vi "MM6.ProcCases.vi"(0 "i ref in":refnum<vi>, 1 "selector":string, 2 "Data":T1, 3 "call cluster":T3={"Object"="", "Selector"="", "CallType"=enum."synchronous", "Async Object"="", "Async Selector"="", "Data Descriptor"="", "Data"=[], "Error #"=0, "Expire"=0}, 5 "error in (no error)":errorcluster) -> (14 "i ref out":refnum<vi>, 17 "answer cluster":T3={"Object"="", "Selector"="", "CallType"=enum."synchronous", "Async Object"="", "Async Selector"="", "Data Descriptor"="", "Data"=[], "Error #"=0, "Expire"=0}, 19 "error out":errorcluster)   [LabVIEW 2014, in "MM6.lvlib"]
doc: "This method is called by a process from within the default case in the event loop. The methods of a class that are linked to events will be called from THIS method. Add your code here."
uses:
  MM6.lvlib
  CS_Core/CSSystem/CoreDefs/CoreDefs.call_type.ctl
  CS_Core/BaseProcess/BaseProcess.descriptor string definition.ctl
  CS_Core/CSSystem/CoreDefs/CoreDefs.rawDataType.ctl
  MM6.status.ctl
  CS_Core/CSSystem/CoreLib/CoreLib.byte array 2 string.vi
  CS_Core/CSSystem/CoreLib/CoreLib.string 2 byte array.vi
  CS_Core/BaseProcess/BaseProcess.lvlib
  CS_Core/CSSystem/CoreLib/CoreLib.lvlib
  CS_Core/CSSystem/CSSystemLib/CSSystemLib.lvlib
  CSlibraries-extern/DimLVEvent/LVDimInterface/LVDimInterface.lvlib
panel:
  in  "MMStatus":T2=enum."config"
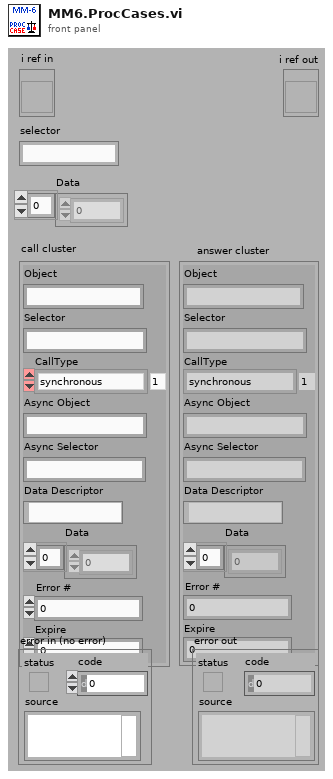
[diagram p1: front panel]
types:
  T1 = typedef "CoreDefs.rawDataType.ctl" = i8[]
  T2 = typedef "MM6.lvlib/MM6.status.ctl" = enum16{"loaded", "load_error", "config", "config_error", "init", "init_error", "data_reset", "data_reset_error", "running", "start_error", "run_error", "abort_requested", "aborted", "stop_requested", "stopped", "stop_error", "Connected", "NOTConnected"}
  T3 = typedef "CoreDefs.call_type.ctl" = cluster{"Object":string, "Selector":string, "CallType":enum16{"simple", "synchronous", "asynchronous"}, "Async Object":string, "Async Selector":string, "Data Descriptor":T4, "Data":T1, "Error #":i32, "Expire":u32}
  T4 = typedef "BaseProcess.lvlib/BaseProcess.descriptor string definition.ctl" = string
  T5 = typedef "MM6.lvlib/MM6.i attribute.ctl" = cluster{"ConfigData":T6, "UsedObjs":string[], "ActScanStep":i32[], "AbortRequest":bool, "StopRequest":bool, "# cycles":i32, "Connected":bool, "MMStatus":T2, "# data":i32, "DIMServices":cluster{"MM6StatusString":string, "MM6StatusID":i32, "discArchiver":string, "discArchiverID":i32, "eventBuilder":string, "eventBuilderID":i32, "GUIIDString":string, "GUIIDStringID":i32}, "dataFile":string, "ExtraDataSets":T21, "PGRunning":T22}
  T6 = typedef "LEBITDefs.lvlib/LEBITDefs.ConfigData.ctl" = cluster{"GenConfig":T7, "Configs":T9[]}
  T7 = typedef "LEBITDefs.lvlib/LEBITDefs.GenConfig.ctl" = cluster{"Mode":i32, "Logs":T8[]}
  T8 = typedef "LEBITDefs.lvlib/LEBITDefs.Log.ctl" = cluster{"Name":string, "FctName":string, "Special":string}
  T9 = typedef "LEBITDefs.lvlib/LEBITDefs.OneConfig.ctl" = cluster{"MCA":T10, "Timing":T11, "Scans":T14[], "FreqDevs":T15[], "CleanDev":T16, "NrCycles":i32, "Specials":T18[], "Delays":T19[], "DAC":T20}
  T10 = typedef "LEBITDefs.lvlib/LEBITDefs.MCA.ctl" = cluster{"Name":string, "Address":string, "NrChannels":i32, "Gate":i32, "NrPipse":i32}
  T11 = typedef "LEBITDefs.lvlib/LEBITDefs.Timing.ctl" = cluster{"TimeTables":cluster{"TimeTable":T12}[], "Memories":T13[], "ScanX":string, "ScanY":string}
  T12 = typedef "LEBITDefs.lvlib/LEBITDefs.Timetable.ctl" = dbl[]
  T13 = typedef "LEBITDefs.lvlib/LEBITDefs.Memory.ctl" = cluster{"Device":string, "ExtTrig":bool, "TT2Use":i32, "PatternTable":string[]}
  T14 = typedef "LEBITDefs.lvlib/LEBITDefs.ScanDev.ctl" = cluster{"Name":string, "FctName":string, "Values":dbl[], "NrScanVals":i32, "Special":string}
  T15 = typedef "LEBITDefs.lvlib/LEBITDefs.FreqDev.ctl" = cluster{"Name":string, "Amp":dbl, "CenterFreq":dbl, "Time":dbl}
  T16 = typedef "LEBITDefs.lvlib/LEBITDefs.CleanDev.ctl" = cluster{"Name":string, "CleanData":T17[]}
  T17 = typedef "LEBITDefs.lvlib/LEBITDefs.CleanDataType.ctl" = cluster{"Amp":dbl, "Center":dbl, "Plus":dbl, "Minus":dbl, "Time":dbl}
  T18 = typedef "LEBITDefs.lvlib/LEBITDefs.Special.ctl" = cluster{"Name":string, "FctName":string, "VerySpecial":string, "Data":dbl}
  T19 = typedef "LEBITDefs.lvlib/LEBITDefs.Delay.ctl" = cluster{"Name":string, "Delay":dbl}
  T20 = typedef "LEBITDefs.lvlib/LEBITDefs.DAC.ctl" = cluster{"Name":string, "Step1":i32, "Step2":i32}
  T21 = typedef "LEBITDefs.lvlib/LEBITDefs.ExtraData.ctl" = cluster{"Ions":cluster{"ExcitIonMass":string, "ExcitIonCharge":i32, "CleanIons":cluster{"CleanIonMass":string, "CleanIonCharge":i32}[]}, "TimingDescription":cluster{"TimeTableDescription":cluster{"Times":string[]}[], "PatternTableDescription":cluster{"Pattern":string[]}[]}, "ScanUnits":string[]}[]
  T22 = typedef "PPG_ABC.lvlib/PPG_ABC.PG_Running.ctl" = i32
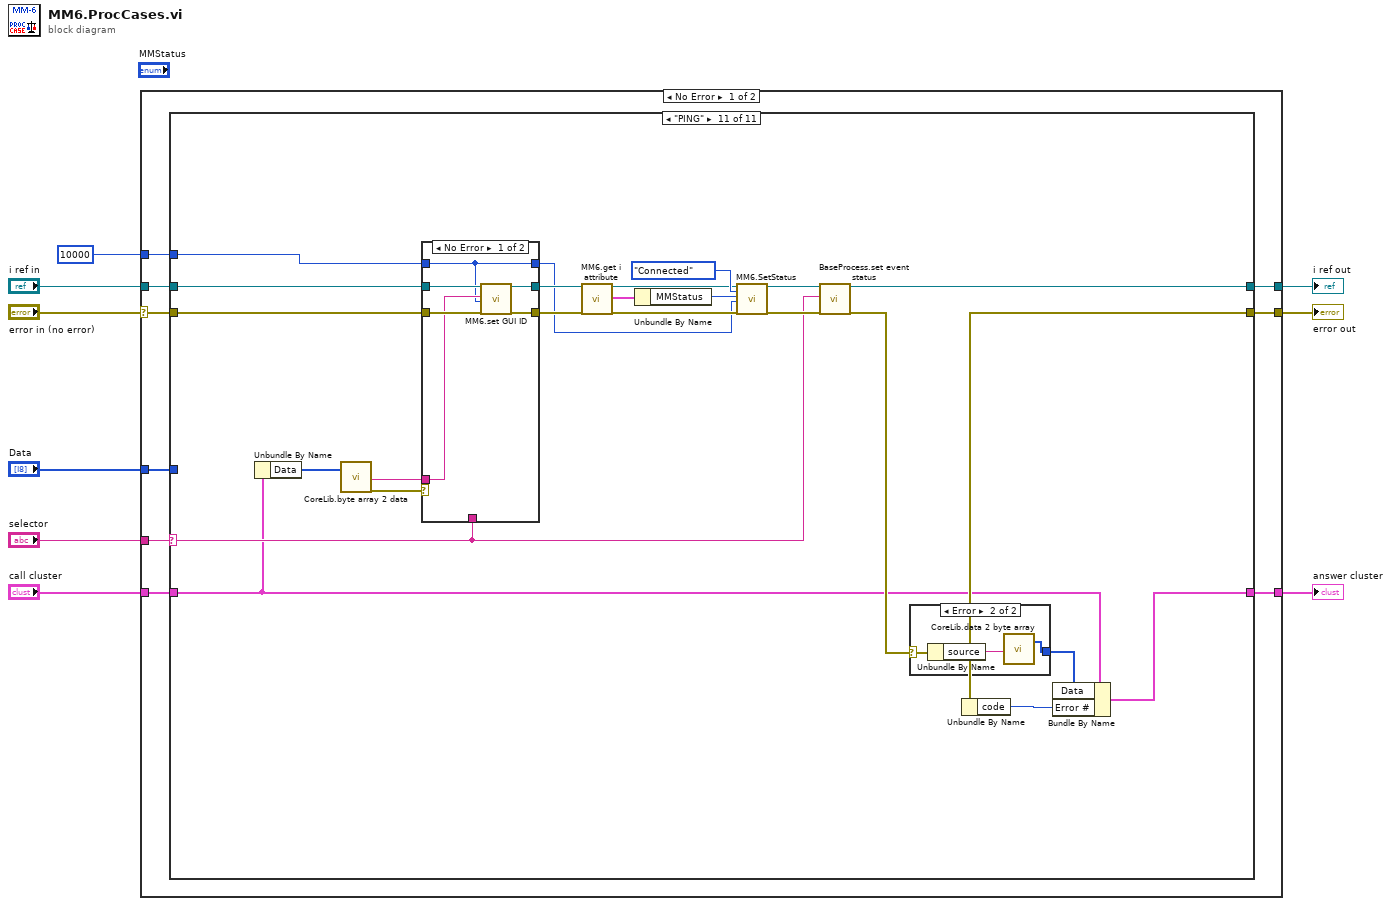
[diagram p0: block diagram]
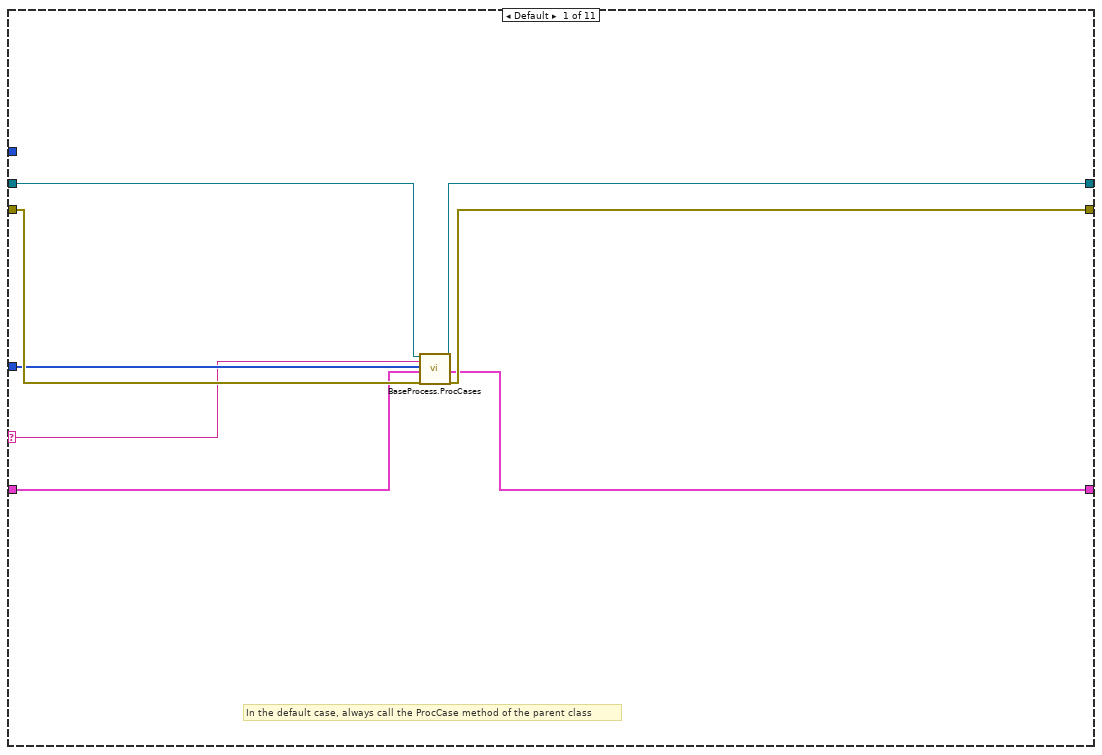
[diagram p2: hidden frame]
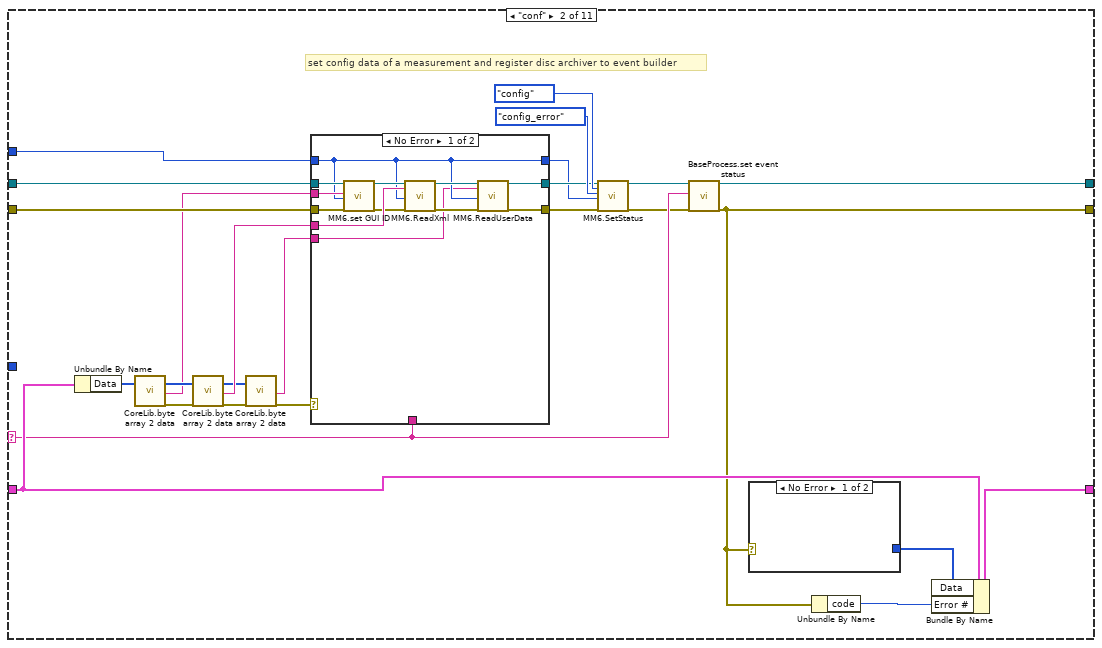
[diagram p3: hidden frame]
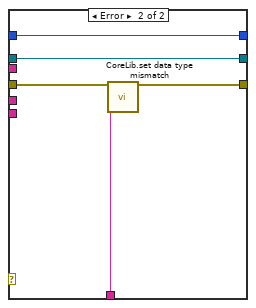
[diagram p4: hidden frame]
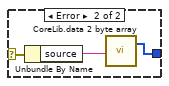
[diagram p5: hidden frame]
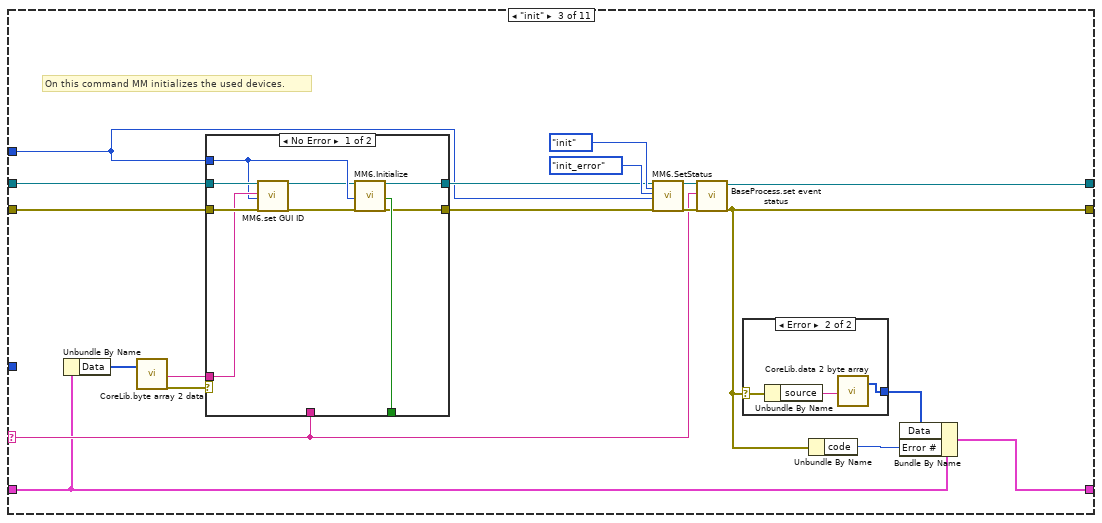
[diagram p6: hidden frame]
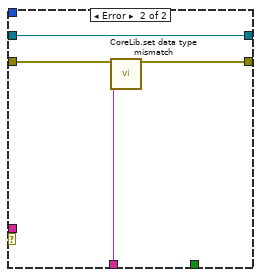
[diagram p7: hidden frame]
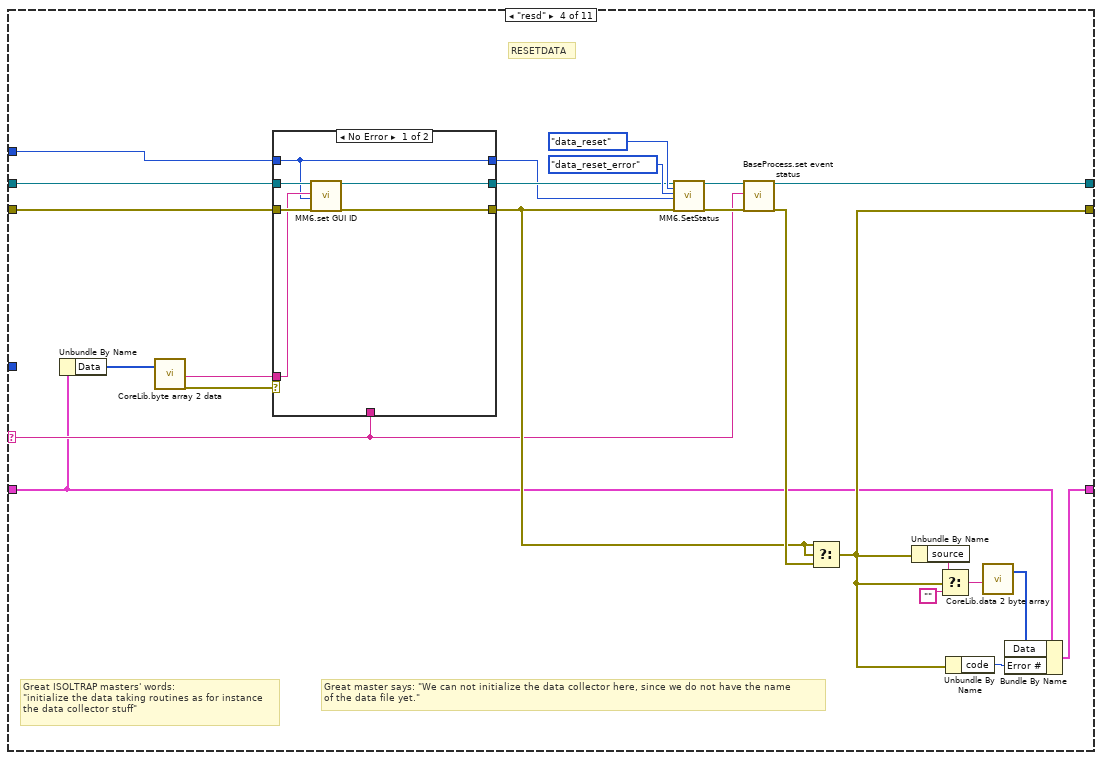
[diagram p9: hidden frame]
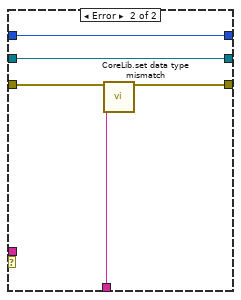
[diagram p10: hidden frame]
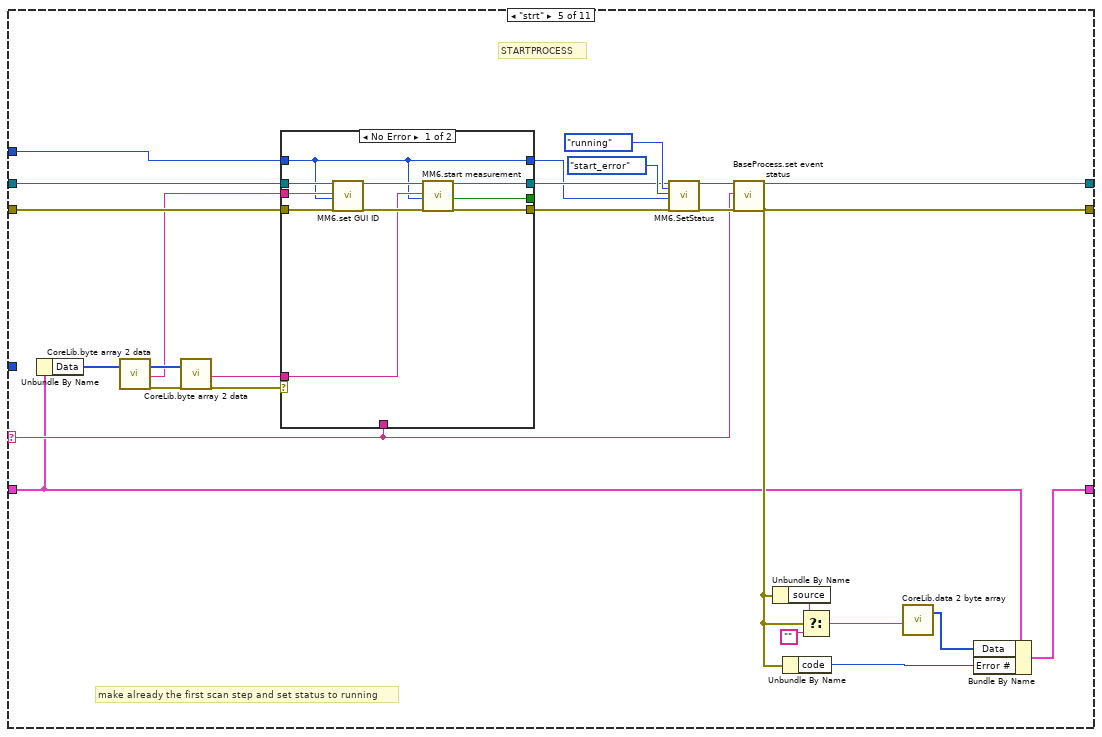
[diagram p11: hidden frame]
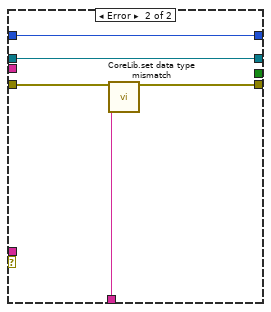
[diagram p12: hidden frame]
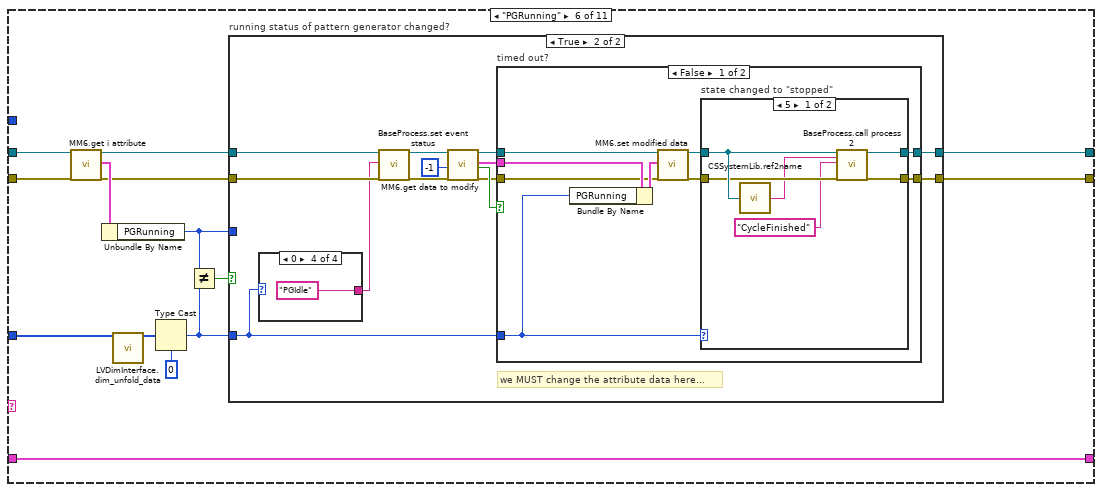
[diagram p13: hidden frame]
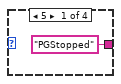
[diagram p15: hidden frame]
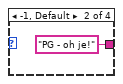
[diagram p16: hidden frame]
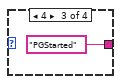
[diagram p17: hidden frame]
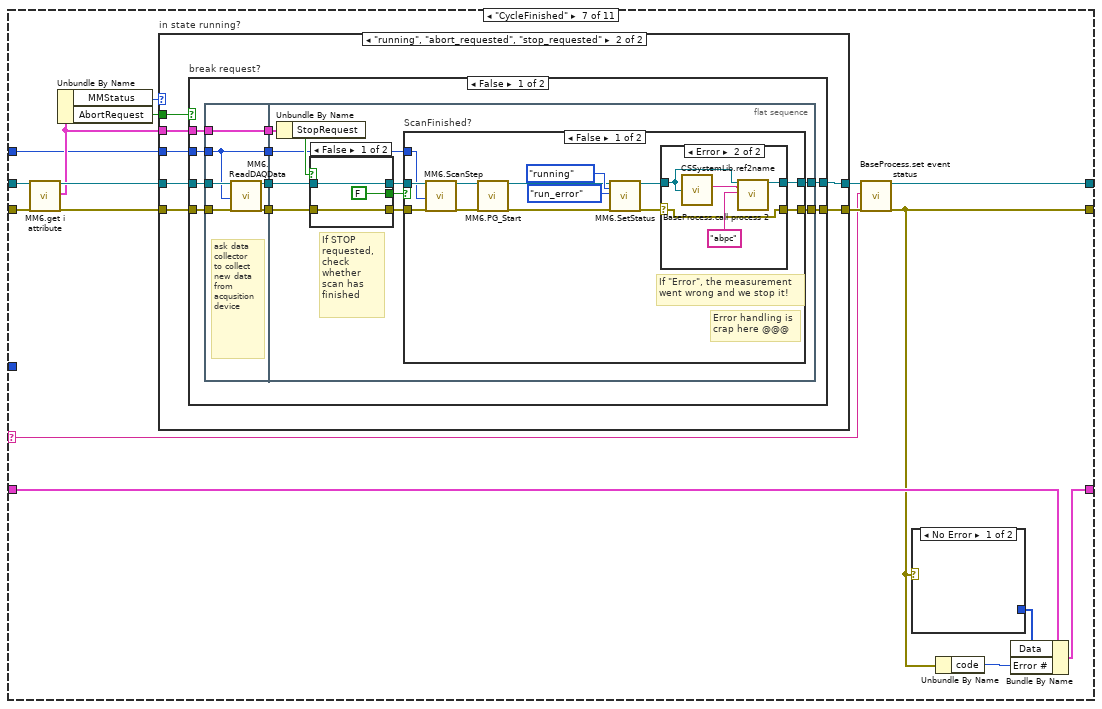
[diagram p20: hidden frame]
diagram:
  n1 = case shown="No Error" "error in (no error)" {
    selector: "error in (no error)" -> [w10 w527]
    tunnel: [w18 w528] -> w9
    tunnel: "call cluster" -> [w17 w528]
    tunnel: [w16 w529] -> w7
    tunnel: [w15 w527] -> w6
    tunnel: "i ref in" -> [w14 w529]
    tunnel: "selector" -> [w13 _]
    tunnel: 10000 ("ms timeout (100)") -> [w12 _]
    tunnel: "Data" -> [w11 _]
    frame No Error {
      n2 = case shown="\"PING\"" w13 {
        selector: w13 -> [w20 w46 w75 w113 w148 _ w237 w338 w398 w450 w492]
        tunnel: w11 -> [w21 _ _ _ _ w197 _ _ _ _ _]
        tunnel: [w26 w41 w81 w129 w168 w186 w241 w354 w413 w469 w512] -> w16
        tunnel: w17 -> [w22 w50 w73 w109 w143 w187 w248 w337 w397 w449 w491]
        tunnel: [w23 w49 w91 w130 w166 w187 w247 w355 w414 w467 w510] -> w18
        tunnel: w10 -> [w25 w32 w78 w114 w153 w193 w251 w358 w417 w454 w497]
        tunnel: [w24 w48 w90 w125 w163 w188 w240 w353 w412 w468 w511] -> w15
        tunnel: w12 -> [_ w36 w80 w112 w151 _ w238 w342 w402 w453 w494]
        tunnel: w14 -> [w19 w33 w79 w116 w155 w194 w252 w359 w418 w455 w500]
        frame Default {
          # "In the default case, always call the ProcCase method of the parent class"
          n3 = call "BaseProcess.ProcCases.vi"("i ref in"=w19, "selector"=w20, "Data"=w21, "call cluster"=w22, "error in (no error)"=w25) -> ("i ref out"=w26:refnum<vi>, "answer cluster"=w23:T3, "error out"=w24:errorcluster)  [unwired: 12 in]
        }
        frame "conf" {
          # "set config data of a measurement and register disc archiver to event builder"
          n4 = Unbundle By Name(w50) -> ("Data"=w47:T1)
          n5 = call-poly "CoreLib.byte array 2 data.vi"("byteArray"=w47) -> ("byteArray out"=w40:T1, "string"=w31:string, "error out"=w39:errorcluster)  [unwired: 16 in]
          n6 = call-poly "CoreLib.byte array 2 data.vi"("byteArray"=w40, "error in (no error)"=w39) -> ("byteArray out"=w29:T1, "string"=w34:string, "error out"=w30:errorcluster)  [unwired: 15 in]
          n7 = call-poly "CoreLib.byte array 2 data.vi"("byteArray"=w29, "error in (no error)"=w30) -> ("string"=w28:string, "error out"=w27:errorcluster)  [unwired: 15 in, 1 out]
          n8 = case shown="No Error" w27 {
            tunnel: [w55 w68] -> w42
            tunnel: w46 -> [_ w69]
            tunnel: w32 -> [w62 w67]
            tunnel: w33 -> [w63 w66]
            tunnel: [w56 w66] -> w37
            tunnel: w36 -> [w54 w65]
            tunnel: [w54 w65] -> w35
            tunnel: w34 -> [w64 _]
            tunnel: w31 -> [w61 _]
            tunnel: w28 -> [w53 _]
            frame No Error {
              n9 = call "MM6.set GUI ID.vi"("i ref in"=w63, "GUIDString"=w61, "ms timeout (10000)"=w54, "error in (no error)"=w62) -> ("i ref out"=w60:refnum<vi>, "error out"=w59:errorcluster)  [unwired: 13 in, 1 out]
              n10 = call "MM6.ReadXml.vi"("i ref in"=w60, "Data"=w64, "timeout ms"=w54, "error in (no error)"=w59) -> ("i ref out"=w58:refnum<vi>, "error out"=w57:errorcluster)  [unwired: 13 in, 1 out]
              n11 = call "MM6.ReadUserData.vi"("i ref in"=w58, "Data"=w53, "timeout ms"=w54, "error in (no error)"=w57) -> ("i ref out"=w56:refnum<vi>, "error out"=w55:errorcluster)  [unwired: 13 in, 1 out]
            }
            frame Error {
              n12 = call "CoreLib.set data type mismatch.vi"("error in (no error)"=w67, "error source"=w69) -> ("error out"=w68:errorcluster)  [unwired: 17 in]
            }
          }
          n13 = call "MM6.SetStatus.vi"("i ref in"=w37, "MMStatusSuccess"=MM6.status."config" ("MMStatus"), "MMStatusFail"=MM6.status."config_error" ("MMStatus"), "ms timeout (10000)"=w35, "error in (no error)"=w42) -> ("i ref out"=w44:refnum<vi>, "error out"=w43:errorcluster)  [unwired: 11 in, 2 out]
          n14 = call "BaseProcess.set event status.vi"("i ref in"=w44, "EventStatus"=w46, "error in (no error)"=w43) -> ("i ref out"=w41:refnum<vi>, "error out"=w48:errorcluster)  [unwired: 14 in, 1 out]
          n15 = case shown="No Error" w48 {
            selector: w48 -> [_ w72]
            tunnel: [_ w71] -> w52
            frame No Error {
            }
            frame Error {
              n16 = Unbundle By Name(w72) -> ("source"=w70:string)
              n17 = call-poly "CoreLib.data 2 byte array.vi"("string"=w70) -> ("byteArray out"=w71:T1)  [unwired: 18 in]
            }
          }
          n18 = Unbundle By Name(w48) -> ("code"=w51:i32)
          n19 = Bundle By Name(cluster=w50, "Data"=w52, "Error #"=w51) -> (w49:T3)
        }
        frame "init" {
          # "On this command MM initializes the used devices."
          n20 = Unbundle By Name(w73) -> ("Data"=w74:T1)
          n21 = call-poly "CoreLib.byte array 2 data.vi"("byteArray"=w74) -> ("string"=w76:string, "error out"=w77:errorcluster)  [unwired: 16 in, 1 out]
          n22 = case shown="No Error" w77 {
            tunnel: [w100 _] -> _
            tunnel: [w99 w103] -> w85
            tunnel: [w98 w102] -> w84
            tunnel: w80 -> [w94 _]
            tunnel: w79 -> [w97 w102]
            tunnel: w78 -> [w96 w104]
            tunnel: w76 -> [w95 _]
            tunnel: w75 -> [_ w101]
            frame No Error {
              n23 = call "MM6.set GUI ID.vi"("i ref in"=w97, "GUIDString"=w95, "ms timeout (10000)"=w94, "error in (no error)"=w96) -> ("i ref out"=w93:refnum<vi>, "error out"=w92:errorcluster)  [unwired: 13 in, 1 out]
              n24 = call "MM6.Initialize.vi"("i ref in"=w93, "ms timeout (10000)"=w94, "error in (no error)"=w92) -> ("i ref out"=w98:refnum<vi>, "timed out"=w100:bool, "error out"=w99:errorcluster)  [unwired: 14 in]
            }
            frame Error {
              n25 = call "CoreLib.set data type mismatch.vi"("error in (no error)"=w104, "error source"=w101) -> ("error out"=w103:errorcluster)  [unwired: 17 in]
            }
          }
          n26 = call "MM6.SetStatus.vi"("i ref in"=w84, "MMStatusSuccess"=MM6.status."init" ("MMStatus"), "MMStatusFail"=MM6.status."init_error" ("MMStatus"), "ms timeout (10000)"=w80, "error in (no error)"=w85) -> ("i ref out"=w83:refnum<vi>, "error out"=w82:errorcluster)  [unwired: 11 in, 2 out]
          n27 = call "BaseProcess.set event status.vi"("i ref in"=w83, "EventStatus"=w75, "error in (no error)"=w82) -> ("i ref out"=w81:refnum<vi>, "error out"=w90:errorcluster)  [unwired: 14 in, 1 out]
          n28 = case shown="Error" w90 {
            selector: w90 -> [_ w107]
            tunnel: [_ w105] -> w89
            frame No Error {
            }
            frame Error {
              n29 = Unbundle By Name(w107) -> ("source"=w106:string)
              n30 = call-poly "CoreLib.data 2 byte array.vi"("string"=w106) -> ("byteArray out"=w105:T1)  [unwired: 18 in]
            }
          }
          n31 = Unbundle By Name(w90) -> ("code"=w88:i32)
          n32 = Bundle By Name(cluster=w73, "Data"=w89, "Error #"=w88) -> (w91:T3)
        }
        frame "resd" {
          # "Great master says: \"We can not initialize the data collector here, since we do not have the name\nof the data file yet.\""
          # "RESETDATA"
          # "Great ISOLTRAP masters' words:\n\"initialize the data taking routines as for instance\nthe data collector stuff\""
          n33 = Unbundle By Name(w109) -> ("Data"=w108:T1)
          n34 = call-poly "CoreLib.byte array 2 data.vi"("byteArray"=w108) -> ("string"=w110:string, "error out"=w115:errorcluster)  [unwired: 16 in, 1 out]
          n35 = case shown="No Error" w115 {
            tunnel: [w133 w139] -> w118
            tunnel: [w132 w141] -> w117
            tunnel: w116 -> [w137 w139]
            tunnel: w114 -> [w136 w142]
            tunnel: w113 -> [_ w140]
            tunnel: w112 -> [w134 w138]
            tunnel: [w134 w138] -> w111
            tunnel: w110 -> [w135 _]
            frame No Error {
              n36 = call "MM6.set GUI ID.vi"("i ref in"=w137, "GUIDString"=w135, "ms timeout (10000)"=w134, "error in (no error)"=w136) -> ("i ref out"=w133:refnum<vi>, "error out"=w132:errorcluster)  [unwired: 13 in, 1 out]
            }
            frame Error {
              n37 = call "CoreLib.set data type mismatch.vi"("error in (no error)"=w142, "error source"=w140) -> ("error out"=w141:errorcluster)  [unwired: 17 in]
            }
          }
          n38 = call "MM6.SetStatus.vi"("i ref in"=w118, "MMStatusSuccess"=MM6.status."data_reset" ("MMStatus"), "MMStatusFail"=MM6.status."data_reset_error" ("MMStatus"), "ms timeout (10000)"=w111, "error in (no error)"=w117) -> ("i ref out"=w122:refnum<vi>, "error out"=w121:errorcluster)  [unwired: 11 in, 2 out]
          n39 = call "BaseProcess.set event status.vi"("i ref in"=w122, "EventStatus"=w113, "error in (no error)"=w121) -> ("i ref out"=w129:refnum<vi>, "error out"=w128:errorcluster)  [unwired: 14 in, 1 out]
          n40 = Select(t=w117, s=w117, f=w128) -> (s? t:f=w125:errorcluster)
          n41 = Unbundle By Name(w125) -> ("source"=w127:string)
          n42 = Select(t=w127, s=w125, f="") -> (s? t:f=w120:string)
          n43 = Unbundle By Name(w125) -> ("code"=w131:i32)
          n44 = call-poly "CoreLib.data 2 byte array.vi"("string"=w120) -> ("byteArray out"=w119:T1)  [unwired: 18 in]
          n45 = Bundle By Name(cluster=w109, "Data"=w119, "Error #"=w131) -> (w130:T3)
        }
        frame "strt" {
          # "STARTPROCESS"
          # "make already the first scan step and set status to running"
          n46 = Unbundle By Name(w143) -> ("Data"=w144:T1)
          n47 = call-poly "CoreLib.byte array 2 data.vi"("byteArray"=w144) -> ("byteArray out"=w156:T1, "string"=w147:string, "error out"=w145:errorcluster)  [unwired: 16 in]
          n48 = call-poly "CoreLib.byte array 2 data.vi"("byteArray"=w156, "error in (no error)"=w145) -> ("string"=w146:string, "error out"=w150:errorcluster)  [unwired: 15 in, 1 out]
          n49 = case shown="No Error" w150 {
            tunnel: w155 -> [w178 w183]
            tunnel: [w176 w183] -> w154
            tunnel: w153 -> [w175 w182]
            tunnel: [w173 w181] -> w152
            tunnel: w151 -> [w170 w180]
            tunnel: [w170 w180] -> w149
            tunnel: w148 -> [_ w179]
            tunnel: w147 -> [w172 _]
            tunnel: w146 -> [w171 _]
            tunnel: [w169 _] -> _
            frame No Error {
              n50 = call "MM6.set GUI ID.vi"("i ref in"=w178, "GUIDString"=w172, "ms timeout (10000)"=w170, "error in (no error)"=w175) -> ("i ref out"=w177:refnum<vi>, "error out"=w174:errorcluster)  [unwired: 13 in, 1 out]
              n51 = call "MM6.start measurement.vi"("i ref in"=w177, "dataFileName"=w171, "ms timeout (10000)"=w170, "error in (no error)"=w174) -> ("i ref out"=w176:refnum<vi>, "timed out"=w169:bool, "error out"=w173:errorcluster)  [unwired: 13 in]
            }
            frame Error {
              n52 = call "CoreLib.set data type mismatch.vi"("error in (no error)"=w182, "error source"=w179) -> ("error out"=w181:errorcluster)  [unwired: 17 in]
            }
          }
          n53 = call "MM6.SetStatus.vi"("i ref in"=w154, "MMStatusSuccess"=MM6.status."running" ("MMStatus"), "MMStatusFail"=MM6.status."start_error" ("MMStatus"), "ms timeout (10000)"=w149, "error in (no error)"=w152) -> ("i ref out"=w159:refnum<vi>, "error out"=w160:errorcluster)  [unwired: 11 in, 2 out]
          n54 = call "BaseProcess.set event status.vi"("i ref in"=w159, "EventStatus"=w148, "error in (no error)"=w160) -> ("i ref out"=w168:refnum<vi>, "error out"=w163:errorcluster)  [unwired: 14 in, 1 out]
          n55 = Unbundle By Name(w163) -> ("source"=w165:string)
          n56 = Unbundle By Name(w163) -> ("code"=w167:i32)
          n57 = Select(t=w165, s=w163, f="") -> (s? t:f=w157:string)
          n58 = call-poly "CoreLib.data 2 byte array.vi"("string"=w157) -> ("byteArray out"=w158:T1)  [unwired: 18 in]
          n59 = Bundle By Name(cluster=w143, "Data"=w158, "Error #"=w167) -> (w166:T3)
        }
        frame "PGRunning" {
          n60 = call "MM6.get i attribute.vi"("i ref in"=w194, "error in (no error)"=w193) -> ("i ref out"=w190:refnum<vi>, "i attribute"=w192:T5, "error out"=w189:errorcluster)  [unwired: 15 in]
          n61 = Unbundle By Name(w192) -> ("PGRunning"=w185:T22)
          n62 = call "LVDimInterface.dim_unfold_data.vi"("rawData"=w197) -> ("data"=w195:i8[])  [unwired: 15 in, 3 out]
          n63 = Type Cast(type=0, x=w195) -> (*(type *) &x=w184:i32)
          n64 = Not Equal?(x=w185, y=w184) -> (x != y?=w191:bool)
          n65 = case "running status of pattern generator changed?" shown="True" w191 {
            tunnel: w190 -> [w199 w205]
            tunnel: w189 -> [w198 w204]
            tunnel: [w198 w206] -> w188
            tunnel: [w199 w207] -> w186
            tunnel: w185 -> [_ _]
            tunnel: w184 -> [_ w201]
            frame False {
            }
            frame True {
              # "we MUST change the attribute data here..."
              n66 = case shown="0" w201 {
                tunnel: ["PGStopped" "PG - oh je!" "PGStarted" "PGIdle"] -> w200
                frame 5 {
                }
                frame -1, Default {
                }
                frame 4 {
                }
                frame 0 {
                }
              }
              n67 = call "BaseProcess.set event status.vi"("i ref in"=w205, "EventStatus"=w200, "error in (no error)"=w204) -> ("i ref out"=w203:refnum<vi>, "error out"=w202:errorcluster)  [unwired: 14 in, 1 out]
              n68 = call "MM6.get data to modify.vi"("i ref in"=w203, "ms timeout (10000)"=-1, "error in (no error)"=w202) -> ("i ref out"=w209:refnum<vi>, "i attribute"=w208:T5, "timed out"=w212:bool, "error out"=w210:errorcluster)  [unwired: 13 in]
              n69 = case "timed out?" shown="False" w212 {
                tunnel: w210 -> [w219 w234]
                tunnel: w209 -> [w225 w235]
                tunnel: [w217 w235] -> w207
                tunnel: [w218 w234] -> w206
                tunnel: w208 -> [w224 _]
                tunnel: w201 -> [w222 _]
                frame False {
                  n70 = Bundle By Name(cluster=w224, "PGRunning"=w222) -> (w223:T5)
                  n71 = call "MM6.set modified data.vi"("i ref in"=w225, "i attribute"=w223, "error in (no error)"=w219) -> ("i ref out"=w221:refnum<vi>, "error out"=w220:errorcluster)  [unwired: 15 in]
                  n72 = case "state changed to \"stopped\"" shown="5" w222 {
                    tunnel: w221 -> [w231 w233]
                    tunnel: w220 -> [w230 w232]
                    tunnel: [w229 w232] -> w218
                    tunnel: [w228 w233] -> w217
                    frame 5 {
                      n73 = call "CSSystemLib.ref2name.vi"("obj refnum"=w231) -> ("name"=w227:string)
                      n74 = call "BaseProcess.call process 2.vi"("i ref in"=w231, "Object"=w227, "Selector"="CycleFinished", "error in (no error)"=w230) -> ("i ref out"=w228:refnum<vi>, "error out"=w229:errorcluster)  [unwired: 14 in]
                    }
                    frame Default {
                    }
                  }
                }
                frame True {
                }
              }
            }
          }
        }
        frame "CycleFinished" {
          n75 = call "MM6.get i attribute.vi"("i ref in"=w252, "error in (no error)"=w251) -> ("i ref out"=w246:refnum<vi>, "i attribute"=w243:T5, "error out"=w245:errorcluster)  [unwired: 15 in]
          n76 = Unbundle By Name(w243) -> ("MMStatus"=w236:T2, "AbortRequest"=w244:bool)
          n77 = case "in state running?" shown="\"running\", \"abort_requested\", \"stop_requested\"" w236 {
            tunnel: w246 -> [w254 w261]
            tunnel: w245 -> [w253 w260]
            tunnel: w244 -> [_ w259]
            tunnel: w243 -> [_ w258]
            tunnel: [w254 w257] -> w242
            tunnel: [w253 w256] -> w239
            tunnel: w238 -> [_ w255]
            frame Default {
            }
            frame "running", "abort_requested", "stop_requested" {
              n78 = case "break request?" shown="False" w259 {
                tunnel: [w268 w330] -> w257
                tunnel: w261 -> [w271 w327]
                tunnel: w260 -> [w270 w326]
                tunnel: [w267 w329] -> w256
                tunnel: w258 -> [w269 _]
                tunnel: w255 -> [w266 w328]
                frame False {
                  n79 = flat-sequence {
                    tunnel: w271 -> [w277]
                    tunnel: [w273] -> w265
                    tunnel: w270 -> [w276]
                    tunnel: w269 -> [w275]
                    tunnel: [w275] -> w264
                    tunnel: w266 -> [w272]
                    tunnel: [w272] -> w263
                    tunnel: [w274] -> w262
                    tunnel: w265 -> [w286]
                    tunnel: w264 -> [w287]
                    tunnel: [w279] -> w268
                    tunnel: [w278] -> w267
                    tunnel: w263 -> [w280]
                    tunnel: w262 -> [w285]
                    frame #0 {
                      # "ask data collector\nto collect new data\nfrom acqusition device"
                      n80 = call "MM6.ReadDAQData.vi"("i ref in"=w277, "ms timeout (10000)"=w272, "error in (no error)"=w276) -> ("i ref out"=w273:refnum<vi>, "error out"=w274:errorcluster)  [unwired: 14 in, 1 out]
                    }
                    frame #1 {
                      # "If STOP requested, check whether scan has finished"
                      n81 = Unbundle By Name(w287) -> ("StopRequest"=w284:bool)
                      n82 = case shown="False" w284 {
                        tunnel: w286 -> [w318 w323]
                        tunnel: [FALSE ("ScanFini") w322] -> w283
                        tunnel: [w318 w321] -> w282
                        tunnel: [w317 w320] -> w281
                        tunnel: w285 -> [w317 w319]
                        frame False {
                        }
                        frame True {
                          n83 = call "MM6.IsScanFinished.vi"("i ref in"=w323, "error in (no error)"=w319) -> ("i ref out"=w321:refnum<vi>, "ScanFini"=w322:bool, "error out"=w320:errorcluster)  [unwired: 15 in]
                        }
                      }
                      n84 = case "ScanFinished?" shown="False" w283 {
                        tunnel: [w300 w315] -> w279
                        tunnel: [w299 w314] -> w278
                        tunnel: w282 -> [w298 w309]
                        tunnel: w281 -> [w297 w308]
                        tunnel: w280 -> [w288 _]
                        frame False {
                          # "Error handling is\ncrap here @@@"
                          # "If \"Error\", the measurement\nwent wrong and we stop it!"
                          n85 = call "MM6.ScanStep.vi"("i ref in"=w298, "ms timeout (10000)"=w288, "error in (no error)"=w297) -> ("i ref out"=w296:refnum<vi>, "error out"=w295:errorcluster)  [unwired: 14 in, 1 out]
                          n86 = call "MM6.PG_Start.vi"("i ref in"=w296, "error in (no error)"=w295) -> ("i ref out"=w292:refnum<vi>, "error out"=w291:errorcluster)  [unwired: 16 in]
                          n87 = call "MM6.SetStatus.vi"("i ref in"=w292, "MMStatusSuccess"=MM6.status."running", "MMStatusFail"=MM6.status."run_error", "error in (no error)"=w291) -> ("i ref out"=w289:refnum<vi>, "error out"=w290:errorcluster)  [unwired: 12 in, 2 out]
                          n88 = case shown="Error" w290 {
                            selector: w290 -> [w302 w303]
                            tunnel: [w301 w307] -> w300
                            tunnel: w289 -> [w301 w304]
                            tunnel: [w302 w303] -> w299
                            frame No Error {
                            }
                            frame Error {
                              n89 = call "CSSystemLib.ref2name.vi"("obj refnum"=w304) -> ("name"=w306:string)
                              n90 = call "BaseProcess.call process 2.vi"("i ref in"=w304, "Object"=w306, "Selector"="abpc") -> ("i ref out"=w307:refnum<vi>)  [unwired: 15 in, 1 out]
                            }
                          }
                        }
                        frame True {
                          # "stop cycle controller...\n@@@@@@"
                          # "scan finished"
                          n91 = call "MM6.PG_Stop.vi"("i ref in"=w309, "error in (no error)"=w308) -> ("i ref out"=w312:refnum<vi>, "error out"=w313:errorcluster)  [unwired: 16 in]
                          n92 = call "MM6.SetStatus.vi"("i ref in"=w312, "MMStatusSuccess"=MM6.status."stopped" ("MMStatus"), "MMStatusFail"=MM6.status."stop_error" ("MMStatus"), "error in (no error)"=w313) -> ("i ref out"=w315:refnum<vi>, "error out"=w314:errorcluster)  [unwired: 12 in, 2 out]
                        }
                      }
                    }
                  }
                }
                frame True {
                  # "stop cyclecontroller..."
                  n93 = call "MM6.PG_Stop.vi"("i ref in"=w327, "error in (no error)"=w326) -> ("i ref out"=w324:refnum<vi>, "error out"=w325:errorcluster)  [unwired: 16 in]
                  n94 = call "MM6.SetStatus.vi"("i ref in"=w324, "MMStatusSuccess"=MM6.status."aborted" ("MMStatus"), "MMStatusFail"=MM6.status."stop_error" ("MMStatus"), "ms timeout (10000)"=w328, "error in (no error)"=w325) -> ("i ref out"=w330:refnum<vi>, "error out"=w329:errorcluster)  [unwired: 11 in, 2 out]
                }
              }
            }
          }
          n95 = call "BaseProcess.set event status.vi"("i ref in"=w242, "EventStatus"=w237, "error in (no error)"=w239) -> ("i ref out"=w241:refnum<vi>, "error out"=w240:errorcluster)  [unwired: 14 in, 1 out]
          n96 = case shown="No Error" w240 {
            selector: w240 -> [_ w335]
            tunnel: [_ w333] -> w250
            frame No Error {
            }
            frame Error {
              n97 = Unbundle By Name(w335) -> ("source"=w334:string)
              n98 = call-poly "CoreLib.data 2 byte array.vi"("string"=w334) -> ("byteArray out"=w333:T1)  [unwired: 18 in]
            }
          }
          n99 = Unbundle By Name(w240) -> ("code"=w249:i32)
          n100 = Bundle By Name(cluster=w248, "Data"=w250, "Error #"=w249) -> (w247:T3)
        }
        frame "abpc" {
          # "\"BREAKPROCESS\""
          # "Don't set the status\nhere. We want to\nkeep the status the\nhas occured before\nbreak was requested"
          n101 = Unbundle By Name(w337) -> ("Data"=w336:T1)
          n102 = call-poly "CoreLib.byte array 2 data.vi"("byteArray"=w336) -> ("string"=w339:string, "error out"=w340:errorcluster)  [unwired: 16 in, 1 out]
          n103 = case shown="No Error" w340 {
            tunnel: w359 -> [w365 w381]
            tunnel: w358 -> [w362 w384]
            tunnel: [w369 _] -> _
            tunnel: [w367 w381] -> w350
            tunnel: [w366 w383] -> w349
            tunnel: w342 -> [w360 w385]
            tunnel: [w360 w385] -> w341
            tunnel: w339 -> [w361 _]
            tunnel: w338 -> [_ w382]
            frame No Error {
              n104 = call "MM6.set GUI ID.vi"("i ref in"=w365, "GUIDString"=w361, "ms timeout (10000)"=w360, "error in (no error)"=w362) -> ("i ref out"=w363:refnum<vi>, "error out"=w364:errorcluster)  [unwired: 13 in, 1 out]
              n105 = call "MM6.get data to modify.vi"("i ref in"=w363, "ms timeout (10000)"=w360, "error in (no error)"=w364) -> ("i ref out"=w371:refnum<vi>, "i attribute"=w368:T5, "timed out"=w369:bool, "error out"=w370:errorcluster)  [unwired: 13 in]
              n106 = case "timed out?" shown="False" w369 {
                tunnel: w371 -> [w377 w380]
                tunnel: [w378 w380] -> w367
                tunnel: w370 -> [w376 w379]
                tunnel: [w375 w379] -> w366
                tunnel: w368 -> [w374 _]
                frame False {
                  n107 = Bundle By Name(cluster=w374, "AbortRequest"=TRUE ("BreakRequest")) -> (w373:T5)
                  n108 = call "MM6.set modified data.vi"("i ref in"=w377, "i attribute"=w373, "error in (no error)"=w376) -> ("i ref out"=w378:refnum<vi>, "error out"=w375:errorcluster)  [unwired: 15 in]
                }
                frame True {
                }
              }
            }
            frame Error {
              n109 = call "CoreLib.set data type mismatch.vi"("error in (no error)"=w384, "error source"=w382) -> ("error out"=w383:errorcluster)  [unwired: 17 in]
            }
          }
          n110 = call "MM6.get i attribute.vi"("i ref in"=w350, "error in (no error)"=w349) -> ("i ref out"=w345:refnum<vi>, "i attribute"=w348:T5, "error out"=w346:errorcluster)  [unwired: 15 in]
          n111 = Unbundle By Name(w348) -> ("MMStatus"=w347:T2)
          n112 = call "MM6.SetStatus.vi"("i ref in"=w345, "MMStatusSuccess"=MM6.status."abort_requested" ("MMStatus"), "MMStatusFail"=w347, "ms timeout (10000)"=w341, "error in (no error)"=w346) -> ("i ref out"=w344:refnum<vi>, "error out"=w343:errorcluster)  [unwired: 11 in, 2 out]
          n113 = case shown="True" FALSE ("Case Constant\n(See Context Help)") {
            tunnel: [w387 w392] -> w354
            tunnel: [w386 w391] -> w353
            tunnel: w338 -> [_ w390]
            tunnel: w344 -> [w387 w389]
            tunnel: w343 -> [w386 w388]
            frame False {
            }
            frame True {
              n114 = call "BaseProcess.set event status.vi"("i ref in"=w389, "EventStatus"=w390, "error in (no error)"=w388) -> ("i ref out"=w392:refnum<vi>, "error out"=w391:errorcluster)  [unwired: 14 in, 1 out]
            }
          }
          n115 = case shown="Error" w353 {
            selector: w353 -> [_ w395]
            tunnel: [_ w394] -> w357
            frame No Error {
            }
            frame Error {
              n116 = Unbundle By Name(w395) -> ("source"=w393:string)
              n117 = call-poly "CoreLib.data 2 byte array.vi"("string"=w393) -> ("byteArray out"=w394:T1)  [unwired: 18 in]
            }
          }
          n118 = Unbundle By Name(w353) -> ("code"=w356:i32)
          n119 = Bundle By Name(cluster=w337, "Data"=w357, "Error #"=w356) -> (w355:T3)
        }
        frame "stop" {
          # "\"STOPPROCESS\""
          n120 = Unbundle By Name(w397) -> ("Data"=w396:T1)
          n121 = call-poly "CoreLib.byte array 2 data.vi"("byteArray"=w396) -> ("string"=w399:string, "error out"=w400:errorcluster)  [unwired: 16 in, 1 out]
          n122 = case shown="No Error" w400 {
            tunnel: w418 -> [w424 w440]
            tunnel: w417 -> [w421 w443]
            tunnel: [w428 _] -> _
            tunnel: [w426 w440] -> w410
            tunnel: [w425 w442] -> w409
            tunnel: w402 -> [w419 w444]
            tunnel: [w419 w444] -> w401
            tunnel: w399 -> [w420 _]
            tunnel: w398 -> [_ w441]
            frame No Error {
              n123 = call "MM6.set GUI ID.vi"("i ref in"=w424, "GUIDString"=w420, "ms timeout (10000)"=w419, "error in (no error)"=w421) -> ("i ref out"=w422:refnum<vi>, "error out"=w423:errorcluster)  [unwired: 13 in, 1 out]
              n124 = call "MM6.get data to modify.vi"("i ref in"=w422, "ms timeout (10000)"=w419, "error in (no error)"=w423) -> ("i ref out"=w430:refnum<vi>, "i attribute"=w427:T5, "timed out"=w428:bool, "error out"=w429:errorcluster)  [unwired: 13 in]
              n125 = case "timed out?" shown="False" w428 {
                tunnel: w430 -> [w436 w439]
                tunnel: [w437 w439] -> w426
                tunnel: w429 -> [w435 w438]
                tunnel: [w434 w438] -> w425
                tunnel: w427 -> [w433 _]
                frame False {
                  n126 = Bundle By Name(cluster=w433, "StopRequest"=TRUE ("BreakRequest")) -> (w432:T5)
                  n127 = call "MM6.set modified data.vi"("i ref in"=w436, "i attribute"=w432, "error in (no error)"=w435) -> ("i ref out"=w437:refnum<vi>, "error out"=w434:errorcluster)  [unwired: 15 in]
                }
                frame True {
                }
              }
            }
            frame Error {
              n128 = call "CoreLib.set data type mismatch.vi"("error in (no error)"=w443, "error source"=w441) -> ("error out"=w442:errorcluster)  [unwired: 17 in]
            }
          }
          n129 = call "MM6.get i attribute.vi"("i ref in"=w410, "error in (no error)"=w409) -> ("i ref out"=w405:refnum<vi>, "i attribute"=w408:T5, "error out"=w406:errorcluster)  [unwired: 15 in]
          n130 = Unbundle By Name(w408) -> ("MMStatus"=w407:T2)
          n131 = call "MM6.SetStatus.vi"("i ref in"=w405, "MMStatusSuccess"=MM6.status."stop_requested" ("MMStatus"), "MMStatusFail"=w407, "ms timeout (10000)"=w401, "error in (no error)"=w406) -> ("i ref out"=w404:refnum<vi>, "error out"=w403:errorcluster)  [unwired: 11 in, 2 out]
          n132 = call "BaseProcess.set event status.vi"("i ref in"=w404, "EventStatus"=w398, "error in (no error)"=w403) -> ("i ref out"=w413:refnum<vi>, "error out"=w412:errorcluster)  [unwired: 14 in, 1 out]
          n133 = case shown="Error" w412 {
            selector: w412 -> [_ w447]
            tunnel: [_ w446] -> w416
            frame No Error {
            }
            frame Error {
              n134 = Unbundle By Name(w447) -> ("source"=w445:string)
              n135 = call-poly "CoreLib.data 2 byte array.vi"("string"=w445) -> ("byteArray out"=w446:T1)  [unwired: 18 in]
            }
          }
          n136 = Unbundle By Name(w412) -> ("code"=w415:i32)
          n137 = Bundle By Name(cluster=w397, "Data"=w416, "Error #"=w415) -> (w414:T3)
        }
        frame "quit" {
          n138 = Unbundle By Name(w449) -> ("Data"=w448:T1)
          n139 = call-poly "CoreLib.byte array 2 data.vi"("byteArray"=w448) -> ("string"=w452:string, "error out"=w451:errorcluster)  [unwired: 16 in, 1 out]
          n140 = case shown="No Error" w451 {
            tunnel: [w478 w486] -> w459
            tunnel: [w477 w484] -> w458
            tunnel: w455 -> [w475 w486]
            tunnel: w454 -> [w473 w485]
            tunnel: w453 -> [w472 _]
            tunnel: w452 -> [_ _]
            tunnel: w450 -> [_ w483]
            tunnel: [w470 _] -> _
            frame No Error {
              n141 = call "MM6.set GUI ID.vi"("i ref in"=w475, "GUIDString"="N/A", "ms timeout (10000)"=w472, "error in (no error)"=w473) -> ("i ref out"=w476:refnum<vi>, "timed out"=w470:bool, "error out"=w474:errorcluster)  [unwired: 13 in]
              n142 = call "MM6.get i attribute.vi"("i ref in"=w476, "error in (no error)"=w474) -> ("i ref out"=w482:refnum<vi>, "i attribute"=w480:T5, "error out"=w481:errorcluster)  [unwired: 15 in]
              n143 = Unbundle By Name(w480) -> ("UsedObjs"=w479:string[])
              n144 = call "MM6.UnloadObjs.vi"("i ref in"=w482, "ObjsToUnload"=w479, "error in (no error)"=w481) -> ("i ref out"=w478:refnum<vi>, "error out"=w477:errorcluster)  [unwired: 15 in]
            }
            frame Error {
              n145 = call "CoreLib.set data type mismatch.vi"("error in (no error)"=w485, "error source"=w483) -> ("error out"=w484:errorcluster)  [unwired: 17 in]
            }
          }
          n146 = call "MM6.get i attribute.vi"("i ref in"=w459, "error in (no error)"=w458) -> ("i ref out"=w460:refnum<vi>, "i attribute"=w463:T5, "error out"=w461:errorcluster)  [unwired: 15 in]
          n147 = Unbundle By Name(w463) -> ("MMStatus"=w462:T2)
          n148 = call "MM6.SetStatus.vi"("i ref in"=w460, "MMStatusSuccess"=MM6.status."NOTConnected" ("MMStatus"), "MMStatusFail"=w462, "ms timeout (10000)"=w453, "error in (no error)"=w461) -> ("i ref out"=w457:refnum<vi>, "error out"=w456:errorcluster)  [unwired: 11 in, 2 out]
          n149 = call "BaseProcess.set event status.vi"("i ref in"=w457, "EventStatus"=w450, "error in (no error)"=w456) -> ("i ref out"=w469:refnum<vi>, "error out"=w468:errorcluster)  [unwired: 14 in, 1 out]
          n150 = case shown="No Error" w468 {
            selector: w468 -> [_ w489]
            tunnel: [_ w488] -> w466
            frame No Error {
            }
            frame Error {
              n151 = Unbundle By Name(w489) -> ("source"=w487:string)
              n152 = call-poly "CoreLib.data 2 byte array.vi"("string"=w487) -> ("byteArray out"=w488:T1)  [unwired: 18 in]
            }
          }
          n153 = Unbundle By Name(w468) -> ("code"=w465:i32)
          n154 = Bundle By Name(cluster=w449, "Data"=w466, "Error #"=w465) -> (w467:T3)
        }
        frame "PING" {
          n155 = Unbundle By Name(w491) -> ("Data"=w490:T1)
          n156 = call-poly "CoreLib.byte array 2 data.vi"("byteArray"=w490) -> ("string"=w495:string, "error out"=w496:errorcluster)  [unwired: 16 in, 1 out]
          n157 = case shown="No Error" w496 {
            tunnel: w500 -> [w518 w522]
            tunnel: [w517 w522] -> w499
            tunnel: [w516 w520] -> w498
            tunnel: w497 -> [w515 w521]
            tunnel: w495 -> [w514 _]
            tunnel: w494 -> [w513 w523]
            tunnel: [w513 w523] -> w493
            tunnel: w492 -> [_ w519]
            frame No Error {
              n158 = call "MM6.set GUI ID.vi"("i ref in"=w518, "GUIDString"=w514, "ms timeout (10000)"=w513, "error in (no error)"=w515) -> ("i ref out"=w517:refnum<vi>, "error out"=w516:errorcluster)  [unwired: 13 in, 1 out]
            }
            frame Error {
              n159 = call "CoreLib.set data type mismatch.vi"("error in (no error)"=w521, "error source"=w519) -> ("error out"=w520:errorcluster)  [unwired: 17 in]
            }
          }
          n160 = call "MM6.get i attribute.vi"("i ref in"=w499, "error in (no error)"=w498) -> ("i ref out"=w503:refnum<vi>, "i attribute"=w506:T5, "error out"=w504:errorcluster)  [unwired: 15 in]
          n161 = Unbundle By Name(w506) -> ("MMStatus"=w505:T2)
          n162 = call "MM6.SetStatus.vi"("i ref in"=w503, "MMStatusSuccess"=MM6.status."Connected" ("MMStatus"), "MMStatusFail"=w505, "ms timeout (10000)"=w493, "error in (no error)"=w504) -> ("i ref out"=w502:refnum<vi>, "error out"=w501:errorcluster)  [unwired: 11 in, 2 out]
          n163 = call "BaseProcess.set event status.vi"("i ref in"=w502, "EventStatus"=w492, "error in (no error)"=w501) -> ("i ref out"=w512:refnum<vi>, "error out"=w511:errorcluster)  [unwired: 14 in, 1 out]
          n164 = case shown="Error" w511 {
            selector: w511 -> [_ w526]
            tunnel: [_ w525] -> w509
            frame No Error {
            }
            frame Error {
              n165 = Unbundle By Name(w526) -> ("source"=w524:string)
              n166 = call-poly "CoreLib.data 2 byte array.vi"("string"=w524) -> ("byteArray out"=w525:T1)  [unwired: 18 in]
            }
          }
          n167 = Unbundle By Name(w511) -> ("code"=w508:i32)
          n168 = Bundle By Name(cluster=w491, "Data"=w509, "Error #"=w508) -> (w510:T3)
        }
      }
    }
    frame Error {
    }
  }
  "answer cluster" <- w9
  "i ref out" <- w7
  "error out" <- w6
